vi "Execute.vi"(8 "error in":errorcluster, 11 "Message Step in":refnum<class "Message Step.lvclass">) -> (0 "error out":errorcluster, 1 "Next Step?":bool, 2 "MSG":string, 3 "Message Step out":refnum<class "Message Step.lvclass">)   [LabVIEW 2017, in "Controller.lvlib" / "Message Step.lvclass"]
uses:
  Message Step.lvclass
  Message Step.lvclass/Message Step.ctl
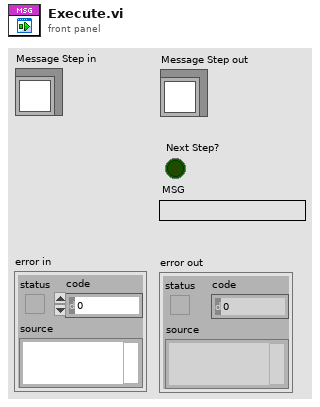
[diagram p1: front panel]
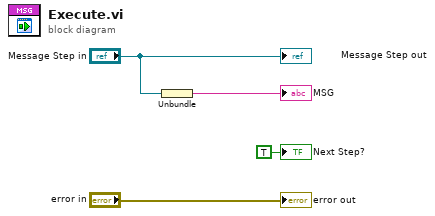
[diagram p0: block diagram]
diagram:
  n1 = Unbundle("Message Step in") -> (→"MSG":string)
  "error out" <- "error in"
  "Message Step out" <- "Message Step in"
  "Next Step?" <- TRUE ("Next Step?")
